vi "GetRef.vi"(8 "error in (no error)":errorcluster, 11 "Progress in":refnum<class "Progress.lvclass">) -> (0 "error out":errorcluster, 2 "ref":refnum<data-value>, 3 "Progress out":refnum<class "Progress.lvclass">)   [LabVIEW 2020, in "Progress.lvlib" / "Progress.lvclass"]
uses:
  Progress.lvclass
  Data.ctl
  Progress.lvclass/Progress.ctl
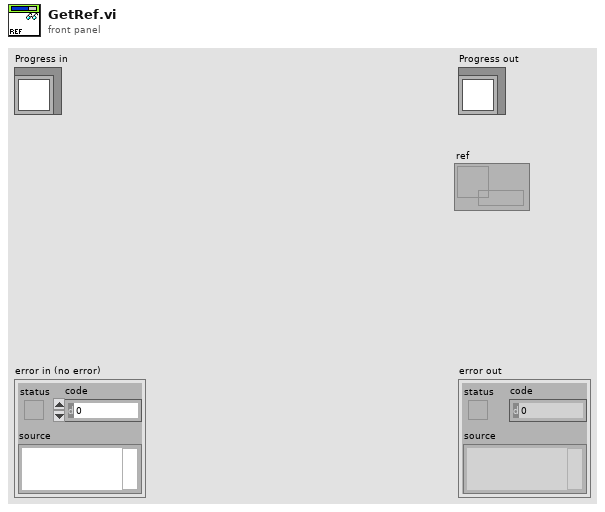
[diagram p1: front panel]
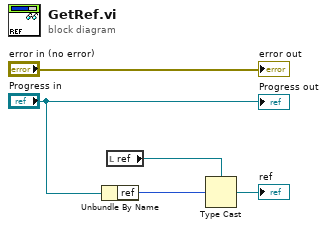
[diagram p0: block diagram]
diagram:
  n1 = Unbundle By Name("Progress in") -> ("ref"=w2:u64)
  n2 = local read "ref"() -> (w3:refnum<data-value>)
  n3 = Type Cast(type=w3, x=w2) -> (*(type *) &x=→"ref":refnum<data-value>)
  "error out" <- "error in (no error)"
  "Progress out" <- "Progress in"
